vi "IOP Control.vi"() -> ()   [LabVIEW 2016]
uses:
  <vilib>/Platform/TimedLoop/XDataNode/timing_clust.ctl
  <vilib>/Platform/TimedLoop/XDataNode/nitl_modes.ctl
  <vilib>/Platform/TimedLoop/XDataNode/wakeup.ctl
  <vilib>/FPGAPlugInAG/PXI-7833R/niLvFpga_Open_PXI-7833R.vi
  <vilib>/Utility/error.llb/Error Cluster From Error Code.vi
  <vilib>/rvi/errors/niLvFpgaAdjustHostInterfaceError.vi
  <vilib>/Utility/file.llb/Write Delimited Spreadsheet (string).vi
  <vilib>/Utility/file.llb/Write Delimited Spreadsheet (DBL).vi
  Subsystems/Global Variables.vi
  <vilib>/FPGAPlugInAG/PXI-7833R/niLvFpga_Reset_PXI-7833R.vi
  <vilib>/FPGAPlugInAG/PXI-7833R/niLvFpga_Close_PXI-7833R.vi
  <vilib>/rvi/interface/nirviOpenFPGA/nirviOpenFPGA.xnode
  FPGA Bitfiles/PhantomControlPI_FPGATarget_QuadCtr2_E2412E44.lvbitx
  IRISS_FPGA_IO.vi
  <vilib>/rvi/interface/nirviReadWriteControl/nirviReadWriteControl.xnode
  <vilib>/platform/TimedLoop/XDataNode/XDataNode.xnode
  <vilib>/rvi/interface/nirviMethod/nirviMethod.xnode
  <vilib>/rvi/interface/nirviCloseFPGA/nirviCloseFPGA.xnode
  <vilib>/Platform/TimedLoop/XDataNode/XDNodeRunTimeDep.lvlib
  Library/KevinLibraryAll/labview2011/kevLib2011.lvlib
  NiFpgaLv.dll
panel:
  out "Pump Period":i32
  in  "Irr Cmd":sgl min=0 max=5 step=0.01 format="%#_4g"
  in  "Tab Control":T1(tab)
  in  "Pump PID Gains":cluster{"Kp":dbl, "Kd":dbl, "Ki":dbl, "Ts":dbl}={"Kp"=0.05, "Kd"=0.01, "Ki"=0.08, "Ts"=0.01}
  in  "Pump Ctrl":bool
  in  "IV Pole PID":cluster{"Kp":dbl, "Kd":dbl, "Ki":dbl, "Ts":dbl}={"Kp"=0.04, "Kd"=0.0, "Ki"=0.03, "Ts"=0.01}
  in  "IV Ctrl":bool
  in  "Pump PD":cluster{"Kp":dbl, "Kd":dbl, "Ki":dbl, "Ts":dbl}={"Kp"=0.001, "Kd"=0.0, "Ki"=0.001, "Ts"=0.01}
  in  "IV Pole PI":cluster{"Kp":dbl, "Kd":dbl, "Ki":dbl, "Ts":dbl}={"Kp"=0.04, "Kd"=0.0, "Ki"=0.03, "Ts"=0.01}
  in  "Dual Stage Ctrl":bool
  in  "Gen Filter":bool
  in  "Cutoff Freq":dbl=5.0 format="%#_13g"
  out "num_LP":dbl[](array[numeric])
  out "num_HP":dbl[](array[numeric])
  in  "Vac PID Gains":cluster{"Kp":dbl, "Kd":dbl, "Ki":dbl, "Ts":dbl}={"Kp"=5.0, "Kd"=0.0, "Ki"=5.0, "Ts"=0.01}
  in  "PID ON/OFF":bool
  in  "OCT Ctrl":bool
  in  "OCT Ctrl PI":cluster{"Kp":dbl, "Kd":dbl, "Ki":dbl, "Ts":dbl}={"Kp"=1.0, "Kd"=0.0, "Ki"=1.0, "Ts"=0.01}
  in  "Irr ON/OFF":bool
  out "Pressure Reading":dbl[](array[numeric]) caption="IOP Output [mmHg]"
  in  "Vacuum Step":bool
  in  "Increase":bool
  in  "Vac Step Size":sgl=50.0 min=0 max=100 step=1 format="%#_13g"
  in  "Wait Time [ms]":i32=200
  in  "Max Limit [mmHg]":dbl=600.0
  in  "Target IOP":sgl=20.0 min=0 max=100 step=1 format="%#_13g"
  out "Vac Input":sgl
  in  "Pump Max":dbl=5.0
  in  "Height":i32
  in  "IV Pole Max":dbl=95.0
  in  "Vac Cmd":sgl min=0 max=100 step=1 format="%#_13g"
  out "Vac Cmd Indicator":dbl
  out "Error(s) Out on Program End":errorcluster
  out "Elaspsed Time":dbl
  in  "File Path":path=path "C:/IOPData1.txt"
  in  "Take Data":bool
  out "File Exists":bool
  in  "Seconds of Data":dbl=30.0
  in  "Prog Stop":bool
  out "I/A and IOP Pressure":T2(graph)
  out "Vac Cmd Chart":sgl(graph)
  # "Irrigation"
  # "Vacuum"
  # "Ant. Chamber"
  # "Vitreous"
  # "Data Saving"
  # "Feedback Control"
  # "1. PID memory release or ramp out\n2. control action direction"
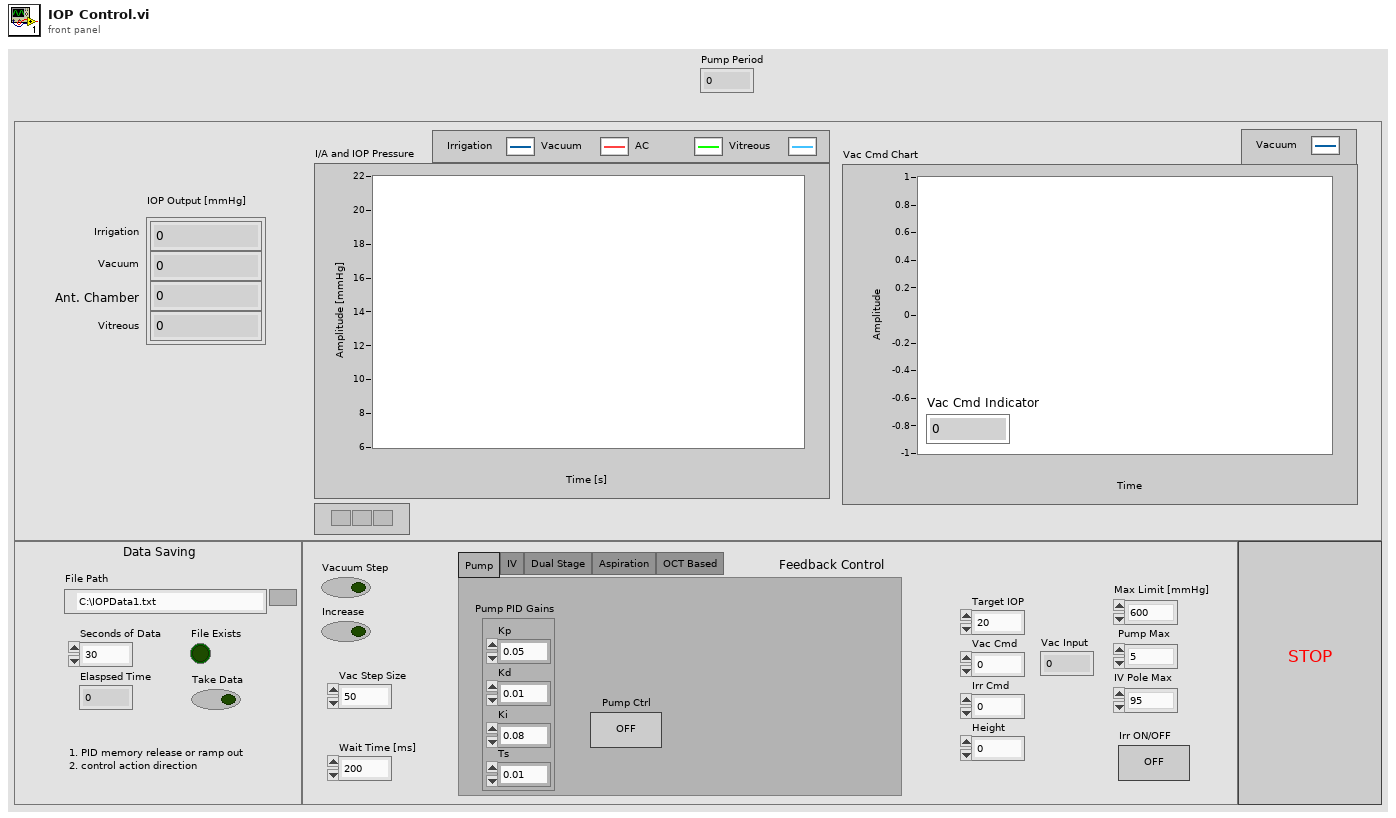
[diagram p1: front panel]
types:
  T1 = enum32{"Pump", "IV", "Dual Stage", "Aspiration", "OCT Based"}
  T2 = cluster{"[0]":dbl, "[1]":dbl, "[2]":dbl, "[3]":dbl, "[4]":dbl, "[5]":dbl, "[6]":dbl, "[7]":dbl, "[8]":dbl}
  T3 = typedef "XDNodeRunTimeDep.lvlib/timing_clust.ctl" = cluster{"Expected End [f-1]":u64, "Actual End [f-1]":u64, "Finished Late? [f-1]":bool, "Expected End [i-1]":u64, "Actual End [i-1]":u64, "Finished Late? [i-1]":bool, "Expected Start [i]":u64, "Actual Start [i]":u64, "Expected Start [f]":u64, "Actual Start [f]":u64, "Source Name":string, "Structure Name":string, "Period":i64, "Deadline":i64, "Offset":i64, "Start":i64, "Priority":i32, "Timeout":i32, "Mode":T4, "Wakeup Reason":T5, "Error":errorcluster, "Source Type":string, "Secondary Source Type":string, "Global End Time":u64, "Global Start Time":u64, "Frame Duration":u64, "Iteration Duration":u64, "Assigned CPU":i32, "I/O Scan Engine Mode":u32}
  T4 = typedef "XDNodeRunTimeDep.lvlib/nitl_modes.ctl" = enum32{"No Change", "Process missed periods, maintain original phase", "Discard missed periods, maintain original phase", "Process missed periods, ignore original phase", "Discard missed periods, ignore original phase"}
  T5 = typedef "XDNodeRunTimeDep.lvlib/wakeup.ctl" = enum32{"Normal", "Aborted", "Asynchronous wakeup", "Timing source error", "Timed loop error", "Timeout"}
  T6 = cluster{"Pressure Reading[0]":dbl, "Pressure Reading[1]":dbl, "Pressure Reading[2]":dbl, "Pressure Reading[3]":dbl, "Pressure Reading[4]":dbl, "Pressure Reading[5]":dbl, "Pressure Reading[6]":dbl, "Pressure Reading[7]":dbl, "Pressure Reading[8]":dbl}
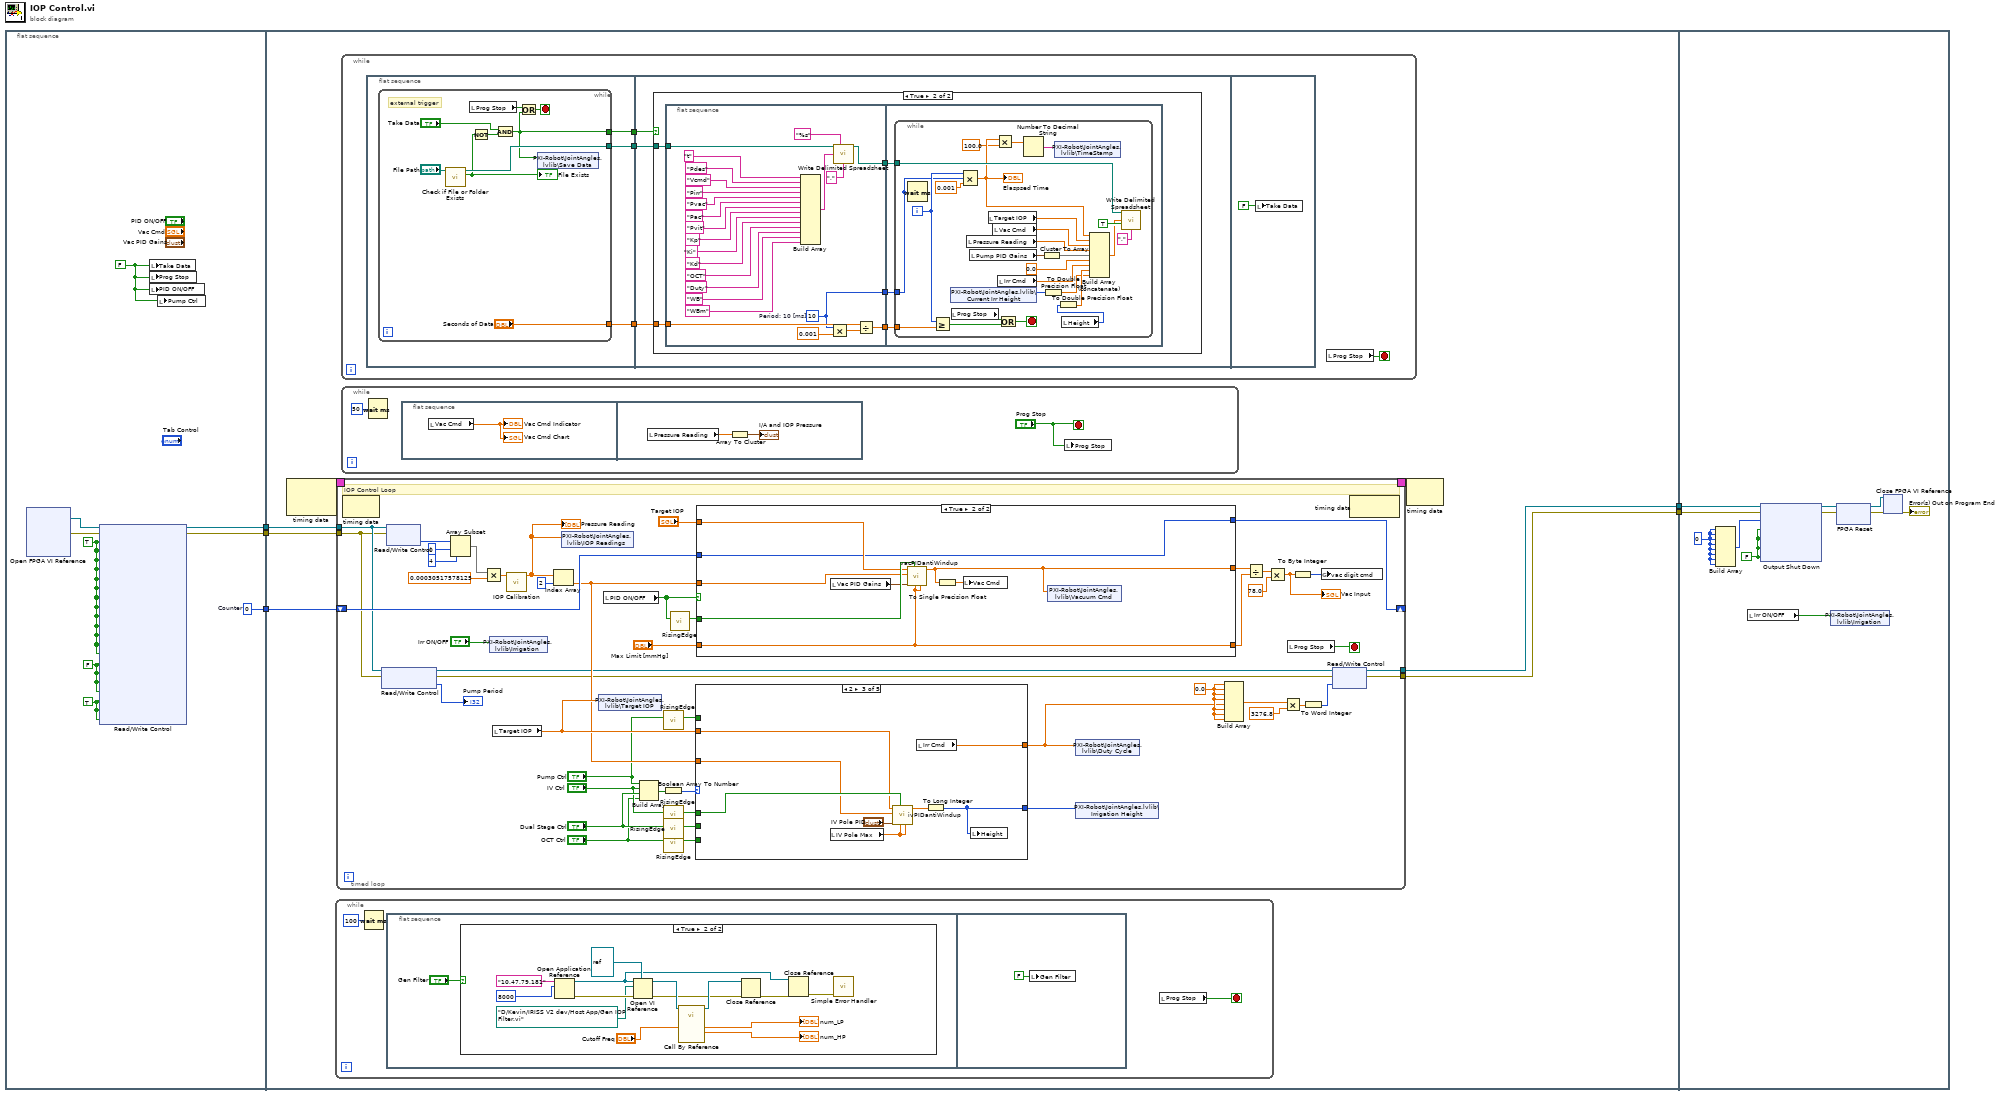
[diagram p0: block diagram]
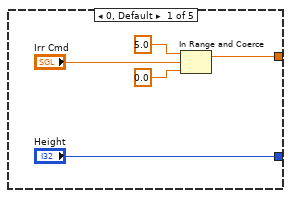
[diagram p3: hidden frame]
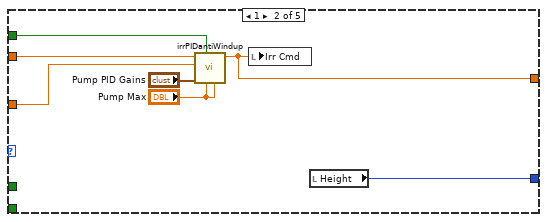
[diagram p4: hidden frame]
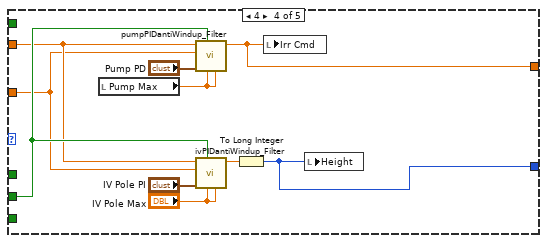
[diagram p5: hidden frame]
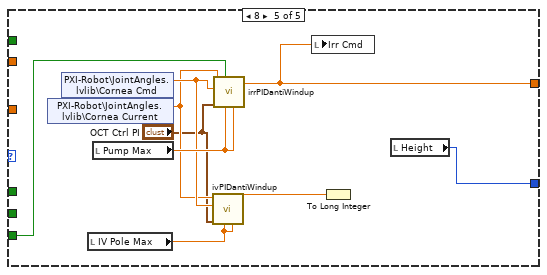
[diagram p6: hidden frame]
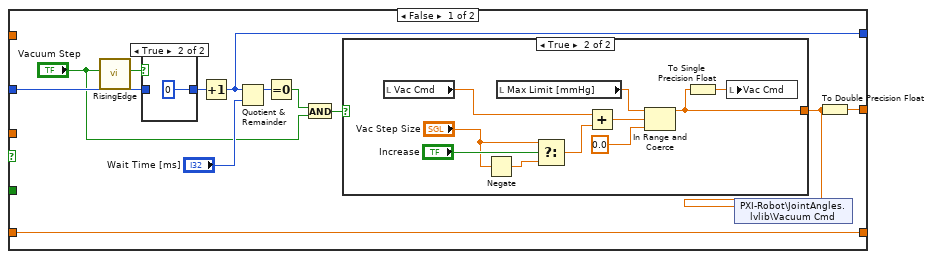
[diagram p7: hidden frame]
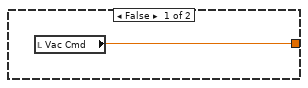
[diagram p9: hidden frame]
diagram:
  n1 = flat-sequence {
    tunnel: [w9] -> w5
    tunnel: [w8] -> w4
    tunnel: [w7] -> w3
    tunnel: w5 -> [w19]
    tunnel: w4 -> [w18]
    tunnel: w3 -> [w17]
    tunnel: [w16] -> w2
    tunnel: [w15] -> w1
    tunnel: w2 -> [w249]
    tunnel: w1 -> [w248]
    frame #0 {
      w7 = 0  # Counter
      w13 = TRUE ("Conn0/DIO12 Button 1")
      w12 = FALSE ("Reset")
      w14 = TRUE ("Reset")
      w6 = FALSE ("stop")
      n2 = xnode "Open FPGA VI Reference"() -> ("FPGA VI Reference Out"=w11:refnum<k20>, "error out"=w10:errorcluster)  [unwired: 2 in]
      n3 = xnode "Read/Write Control"("FPGA VI Reference In"=w11, "error in"=w10, "Reset 1"=w14, "Reset 3"=w14, "Reset 9"=w14, "Reset 10"=w14, "Reset 11"=w14, "Reset 12"=w14, "Reset 13"=w14, "Reset 14"=w14, "Reset 15"=w14, "Reset 16"=w14, "Reset 17"=w14, "Reset C1-1"=w14, "Reset C1-4"=w14, "INHB X"=w12, "INHB Y"=w12, "INHB Z"=w12, "INHB OCT Mot"=w12, "Conn0/DIO12 Button 1"=w13, "Conn0/DIO13 Button 2"=w13, "Conn0/DIO15 Button 4"=w13) -> ("FPGA VI Reference Out"=w9:refnum<k20>, "error out"=w8:errorcluster)
      n4 = local write "Take Data"(w6) -> ()
      n5 = local write "Prog Stop"(w6) -> ()
      n6 = local write "PID ON/OFF"(w6) -> ()
      n7 = local write "Pump Ctrl"(w6) -> ()
    }
    frame #1 {
      n8 = node-c288 ("Input Node")() -> (w21:T3)  [unwired: 2 in]
      n9 = while {
        stop <- w22 stop-if-true
        n10 = Wait (ms)(milliseconds to wait=u32 100) -> ()  [unwired: 1 out]
        n11 = flat-sequence {
          frame #0 {
            n12 = case shown="True" "Gen Filter" {
              frame False {
              }
              frame True {
                n13 = Open Application Reference(10:u16 8000 ("port number or service name (3363)"), 11:"10.47.79.181" ("machine name (\"\":  open local reference)")) -> (0:w33:errorcluster, 3:w35:refnum<vi>)  [unwired: 2 in]
                n14 = Open VI Reference(type specifier VI Refnum (for type only)=refnum<vi> refnum, application reference (local)=w35, vi path=path "D:/Kevin/IRISS V2 dev/Host App/Gen IOP Filter.vi", error in (no error)=w33) -> (vi reference=w30:refnum<vi>, error out=w28:errorcluster)  [unwired: 2 in]
                n15 = call-by-ref "?"(reference=w30, "Cutoff Freq"="Cutoff Freq") -> (reference out=w29:refnum<vi>, "num_HP"=→"num_HP":dbl[], "num_LP"=→"num_LP":dbl[])  [unwired: 10 in, 1 out]
                n16 = Close Reference(reference=w29, error in (no error)=w28) -> (error out=w34:errorcluster)
                n17 = Close Reference(reference=w35, error in (no error)=w34) -> (error out=w32:errorcluster)
                n18 = call <vilib>:"Simple Error Handler.vi"("error in (no error)"=w32) -> ()  [unwired: 4 in, 5 out]
              }
            }
          }
          frame #1 {
            n19 = local write "Gen Filter"(FALSE ("Gen Filter")) -> ()
          }
        }
        n20 = local read "Prog Stop"() -> (w22:bool)
      }
      n21 = timed-loop {
        timing: w21 -> [_]
        timing-out: [_] -> w20
        tunnel: w19 -> [w44]
        tunnel: w18 -> [w42]
        shift-right: [w68] -> _
        shift-left: w17 -> [w69]
        tunnel: [w67] -> w16
        tunnel: [w66] -> w15
        stop <- w79 stop-if-true
        w46 = 0.0 ("lower limit")
        # "IOP Control Loop"
        n22 = node-c288() -> ()  [unwired: 1 in, 1 out]
        n23 = xnode "Read/Write Control"("FPGA VI Reference In"=w44, "error in"=w42) -> ("FPGA VI Reference Out"=w43:refnum<k20>, "error out"=w41:errorcluster, "Pump Period"=→"Pump Period":i32)
        n24 = xnode "Read/Write Control"("FPGA VI Reference In"=w44, "error in"=w42) -> ("AI"=w82:i16[])  [unwired: 2 out]
        n25 = Array Subset(array=w82, index=0, length=4) -> (w87:i16[])
        n26 = Multiply(x=w87, y=0.00030517578125) -> (x*y=w72:dbl[])
        n27 = shared-variable "PXI-Robot\\JointAngles.lvlib\\Irrigation"("Irr ON/OFF") -> ()  [unwired: 1 in, 1 out]
        n28 = local read "Target IOP"() -> (w63:sgl)
        n29 = call "IOP Calibration.vi"("IOP Input [V]"=w72) -> ("IOP Output [mmHg]"=w64:dbl[])  [unwired: 10 in]
        "Pressure Reading" <- w64
        n30 = Index Array(array=w64, index=2) -> (element=w62:dbl)
        n31 = shared-variable "PXI-Robot\\JointAngles.lvlib\\IOP Readings"(w64) -> ()  [unwired: 1 in, 1 out]
        n32 = shared-variable "PXI-Robot\\JointAngles.lvlib\\Target IOP"(w63) -> ()  [unwired: 1 in, 1 out]
        n33 = local read "PID ON/OFF"() -> (w80:bool)
        n34 = Build Array("Pump Ctrl", "IV Ctrl", "Dual Stage Ctrl", "OCT Ctrl") -> (w59:bool[])
        n35 = call "RisingEdge.vi"("Signal In"="Pump Ctrl") -> ("Rising Edge"=w61:bool)  [unwired: 10 in]
        n36 = Boolean Array To Number(Boolean array=w59) -> (number=w60:u32)
        n37 = call "RisingEdge.vi"("Signal In"="IV Ctrl") -> ("Rising Edge"=w53:bool)  [unwired: 10 in]
        n38 = call "RisingEdge.vi"("Signal In"="Dual Stage Ctrl") -> ("Rising Edge"=w57:bool)  [unwired: 10 in]
        n39 = call "RisingEdge.vi"("Signal In"="OCT Ctrl") -> ("Rising Edge"=w51:bool)  [unwired: 10 in]
        n40 = call "RisingEdge.vi"("Signal In"=w80) -> ("Rising Edge"=w81:bool)  [unwired: 10 in]
        n41 = case shown="2" w60 {
          tunnel: w63 -> [_ w97 w106 w113 _]
          tunnel: w62 -> [_ w96 w105 w112 _]
          tunnel: w61 -> [_ w95 _ _ _]
          tunnel: [w88 w93 w100 w108 w118] -> w45
          tunnel: ["Height" w94 w101 w117 w119] -> w56
          tunnel: w57 -> [_ _ _ w114 _]
          tunnel: w53 -> [_ _ w107 _ _]
          tunnel: w51 -> [_ _ _ _ w125]
          frame 0, Default {
            n42 = In Range and Coerce(upper limit=5.0, x="Irr Cmd", lower limit=0.0) -> (coerced(x)=w88:dbl)  [unwired: 1 out]
          }
          frame 1 {
            n43 = call "irrPIDantiWindup.vi"("Saturation U"="Pump Max", "Saturation M"="Pump Max", "Reset"=w95, "PID Gains"="Pump PID Gains", "Feedback"=w96, "Reference"=w97) -> ("Control"=w93:dbl)  [unwired: 5 in]
            n44 = local write "Irr Cmd"(w93) -> ()
            n45 = local read "Height"() -> (w94:i32)
          }
          frame 2 {
            n46 = local read "IV Pole Max"() -> (w103:dbl)
            n47 = call "ivPIDantiWindup.vi"("Saturation U"=w103, "Saturation M"=w103, "Reset"=w107, "PID Gains"="IV Pole PID", "Feedback"=w105, "Reference"=w106) -> ("Control"=w102:dbl)  [unwired: 5 in]
            n48 = local read "Irr Cmd"() -> (w100:sgl)
            n49 = To Long Integer(number=w102) -> (32bit integer=w101:i32)
            n50 = local write "Height"(w101) -> ()
          }
          frame 4 {
            n51 = local read "Pump Max"() -> (w110:dbl)
            n52 = call "pumpPIDantiWindup_Filter.vi"("Saturation U"=w110, "Saturation M"=w110, "Reset"=w114, "PID Gains"="Pump PD", "Feedback"=w112, "Reference"=w113) -> ("Control"=w108:dbl)  [unwired: 5 in]
            n53 = call "ivPIDantiWindup_Filter.vi"("Saturation U"="IV Pole Max", "Saturation M"="IV Pole Max", "Reset"=w114, "PID Gains"="IV Pole PI", "Feedback"=w112, "Reference"=w113) -> ("Control"=w116:dbl)  [unwired: 5 in]
            n54 = To Long Integer(number=w116) -> (32bit integer=w117:i32)
            n55 = local write "Irr Cmd"(w108) -> ()
            n56 = local write "Height"(w117) -> ()
          }
          frame 8 {
            n57 = shared-variable "PXI-Robot\\JointAngles.lvlib\\Cornea Current"() -> (w123:dbl)  [unwired: 1 in, 1 out]
            n58 = shared-variable "PXI-Robot\\JointAngles.lvlib\\Cornea Cmd"() -> (w124:dbl)  [unwired: 1 in, 1 out]
            n59 = local read "IV Pole Max"() -> (w121:dbl)
            n60 = local read "Pump Max"() -> (w126:dbl)
            n61 = call "ivPIDantiWindup.vi"("Saturation U"=w121, "Saturation M"=w121, "PID Gains"="OCT Ctrl PI", "Feedback"=w124, "Reference"=w123) -> ("Control"=w120:dbl)  [unwired: 6 in]
            n62 = call "irrPIDantiWindup.vi"("Saturation U"=w126, "Saturation M"=w126, "Reset"=w125, "PID Gains"="OCT Ctrl PI", "Feedback"=w124, "Reference"=w123) -> ("Control"=w118:dbl)  [unwired: 5 in]
            n63 = local write "Irr Cmd"(w118) -> ()
            n64 = To Long Integer(number=w120) -> ()  [unwired: 1 out]
            n65 = local read "Height"() -> (w119:i32)
          }
        }
        n66 = case shown="True" w80 {
          tunnel: w62 -> [_ w156]
          tunnel: "Target IOP" -> [_ w157]
          tunnel: [w138 w152] -> w78
          tunnel: "Max Limit [mmHg]" -> [w137 w159]
          tunnel: [w137 w159] -> w70
          tunnel: w81 -> [_ w158]
          tunnel: w69 -> [w131 w153]
          tunnel: [w128 w153] -> w68
          frame False {
            n67 = call "RisingEdge.vi"("Signal In"="Vacuum Step") -> ("Rising Edge"=w132:bool)  [unwired: 10 in]
            n68 = case shown="True" w132 {
              tunnel: [w139 0] -> w135
              tunnel: w131 -> [w139 _]
              frame False {
              }
              frame True {
              }
            }
            n69 = Increment(x=w135) -> (x+1=w128:i32)
            n70 = Quotient & Remainder(x=w128, y="Wait Time [ms]") -> (x-y*floor(x/y)=w134:i32)  [unwired: 1 out]
            n71 = Equal To 0?(x=w134) -> (x = 0?=w136:bool)
            n72 = And(x=w136, y="Vacuum Step") -> (x .and. y?=w130:bool)
            n73 = case shown="True" w130 {
              tunnel: [w141 w151] -> w127
              frame False {
                n74 = local read "Vac Cmd"() -> (w141:sgl)
              }
              frame True {
                n75 = local read "Vac Cmd"() -> (w145:sgl)
                n76 = Negate(x="Vac Step Size") -> (-x=w143:sgl)
                n77 = local read "Max Limit [mmHg]"() -> (w148:dbl)
                n78 = Select(t="Vac Step Size", s="Increase", f=w143) -> (s? t:f=w146:sgl)
                n79 = Add(x=w145, y=w146) -> (x+y=w150:sgl)
                n80 = In Range and Coerce(upper limit=w148, x=w150, lower limit=0.0 ("y")) -> (coerced(x)=w151:dbl)  [unwired: 1 out]
                n81 = To Single Precision Float(number=w151) -> (single precision float=w142:sgl)
                n82 = local write "Vac Cmd"(w142) -> ()
              }
            }
            n83 = shared-variable "PXI-Robot\\JointAngles.lvlib\\Vacuum Cmd"(w127) -> ()  [unwired: 1 in, 1 out]
            n84 = To Double Precision Float(number=w127) -> (double precision float=w138:dbl)
          }
          frame True {
            n85 = local read "Vac PID Gains"() -> (w155:cluster{"Kp":dbl, "Kd":dbl, "Ki":dbl, "Ts":dbl})
            n86 = call "vacPIDantiWindup.vi"("Saturation U"=w159, "Saturation M"=w159, "Reset"=w158, "PID Gains"=w155, "Feedback"=w156, "Reference"=w157) -> ("Control"=w152:dbl)  [unwired: 5 in]
            n87 = To Single Precision Float(number=w152) -> (single precision float=w154:sgl)
            n88 = local write "Vac Cmd"(w154) -> ()
            n89 = shared-variable "PXI-Robot\\JointAngles.lvlib\\Vacuum Cmd"(w152) -> ()  [unwired: 1 in, 1 out]
          }
        }
        n90 = shared-variable "PXI-Robot\\JointAngles.lvlib\\Duty Cycle"(w45) -> ()  [unwired: 1 in, 1 out]
        n91 = shared-variable "PXI-Robot\\JointAngles.lvlib\\Irrigation Height"(w56) -> ()  [unwired: 1 in, 1 out]
        n92 = Build Array(w46, w46, w46, w46, w45, w46, w46, w46) -> (w47:dbl[])
        n93 = Divide(x=w78, y=w70) -> (x/y=w77:dbl)
        n94 = Multiply(x=w77, y=78.0) -> (x*y=w71:dbl)
        "Vac Input" <- w71
        n95 = Multiply(x=w47, y=3276.8) -> (x*y=w49:dbl[])
        n96 = local read "Prog Stop"() -> (w79:bool)
        n97 = To Byte Integer(number=w71) -> (8bit integer=w75:i8)
        n98 = To Word Integer(number=w49) -> (16bit integer=w48:i16[])
        n99 = global write "Global Variables.vi" "vac digit cmd"(w75) -> ()
        n100 = xnode "Read/Write Control"("FPGA VI Reference In"=w43, "error in"=w41, "AO"=w48) -> ("FPGA VI Reference Out"=w67:refnum<k20>, "error out"=w66:errorcluster)
        n101 = node-c288() -> ()  [unwired: 1 in, 1 out]
      }
      n102 = while {
        stop <- w169 stop-if-true
        n103 = flat-sequence {
          tunnel: [w173] -> w172
          tunnel: [w175] -> w171
          tunnel: [w174] -> w170
          tunnel: w172 -> [w187]
          tunnel: w171 -> [w186]
          tunnel: w170 -> [w185]
          frame #0 {
            n104 = while {
              tunnel: [w180] -> w175
              tunnel: ["Seconds of Data"] -> w174
              tunnel: [w176] -> w173
              stop <- w184 stop-if-true
              # "external trigger"
              n105 = call <vilib>:"Check if File or Folder Exists.vi"("path"="File Path") -> ("file or folder exists?"=w179:bool, "dup path"=w180:path)  [unwired: 8 in, 1 out]
              "File Exists" <- w179
              n106 = local read "Prog Stop"() -> (w182:bool)
              n107 = Not(x=w179) -> (.not. x?=w178:bool)
              n108 = And(x="Take Data", y=w178) -> (x .and. y?=w176:bool)
              n109 = Or(x=w182, y=w176) -> (x .or. y?=w184:bool)
              n110 = shared-variable "PXI-Robot\\JointAngles.lvlib\\Save Data"(w176) -> ()  [unwired: 1 in, 1 out]
            }
          }
          frame #1 {
            n111 = case shown="True" w187 {
              tunnel: w186 -> [_ w192]
              tunnel: w185 -> [_ w190]
              frame False {
              }
              frame True {
                n112 = flat-sequence {
                  tunnel: w192 -> [w206]
                  tunnel: [w204] -> w191
                  tunnel: w190 -> [w214]
                  tunnel: [w212] -> w189
                  tunnel: [w201] -> w188
                  tunnel: w191 -> [w219]
                  tunnel: w189 -> [w218]
                  tunnel: w188 -> [w217]
                  frame #0 {
                    w201 = 10  # Period: 10 [ms]
                    n113 = Build Array("t" ("delimiter (\\t)"), "Pdes" ("delimiter (\\t)"), "Vcmd" ("delimiter (\\t)"), "Pirr" ("delimiter (\\t)"), "Pvac" ("delimiter (\\t)"), "Pac" ("delimiter (\\t)"), "Pvit" ("delimiter (\\t)"), "Kp" ("delimiter (\\t)"), "Ki" ("delimiter (\\t)"), "Kd" ("delimiter (\\t)"), "OCT" ("delimiter (\\t)"), "Duty" ("delimiter (\\t)"), "WB" ("delimiter (\\t)"), "WBm" ("delimiter (\\t)")) -> (w203:string[])
                    n114 = Multiply(x=w201, y=0.001) -> (x*y=w213:dbl)
                    n115 = call-poly <vilib>:"Write Delimited Spreadsheet.vi"("file path (dialog if empty)"=w206, "format (%s)"="%s", "1D data"=w203, "delimiter (\\t)"="," ("delimiter (\\t)")) -> ("new file path (Not A Path if cancelled)"=w204:path)  [unwired: 10 in, 1 out]
                    n116 = Divide(x=w214, y=w213) -> (x/y=w212:dbl)
                  }
                  frame #1 {
                    n117 = while {
                      tunnel: w219 -> [w239]
                      tunnel: w218 -> [w241]
                      tunnel: w217 -> [w232]
                      i -> [w242]
                      stop <- w244 stop-if-true
                      n118 = Wait (ms)(milliseconds to wait=w232) -> ()  [unwired: 1 out]
                      n119 = Greater Or Equal?(x=w242, y=w241) -> (x >= y?=w240:bool)
                      n120 = shared-variable "PXI-Robot\\JointAngles.lvlib\\Current Irr Height"() -> (w231:i32)  [unwired: 1 in, 1 out]
                      n121 = local read "Prog Stop"() -> (w245:bool)
                      n122 = Compound Arithmetic op=MULTIPLY(w242, w232, 0.001 ("y")) -> (w226:dbl)
                      "Elaspsed Time" <- w226
                      n123 = local read "Pressure Reading"() -> (w233:dbl[])
                      n124 = local read "Pump PID Gains"() -> (w221:cluster{"Kp":dbl, "Kd":dbl, "Ki":dbl, "Ts":dbl})
                      n125 = local read "Target IOP"() -> (w235:sgl)
                      n126 = local read "Vac Cmd"() -> (w234:sgl)
                      n127 = Multiply(x=w226, y=100.0) -> (x*y=w224:dbl)
                      n128 = local read "Irr Cmd"() -> (w222:sgl)
                      n129 = Or(x=w245, y=w240) -> (x .or. y?=w244:bool)
                      n130 = Number To Decimal String(number=w224) -> (decimal integer string=w223:string)  [unwired: 1 in]
                      n131 = Cluster To Array(cluster=w221) -> (array=w220:dbl[])
                      n132 = To Double Precision Float(number=w231) -> (double precision float=w227:dbl)
                      n133 = shared-variable "PXI-Robot\\JointAngles.lvlib\\TimeStamp"(w223) -> ()  [unwired: 1 in, 1 out]
                      n134 = local read "Height"() -> (w229:i32)
                      n135 = To Double Precision Float(number=w229) -> (double precision float=w228:dbl)
                      n136 = Build Array (concatenate)(w226, w235, w234, w233, w220, 0.0 ("y"), w222, w228, w227) -> (w237:dbl[])
                      n137 = call-poly <vilib>:"Write Delimited Spreadsheet.vi"("file path (dialog if empty)"=w239, "1D data"=w237, "append to file? (new file:F)"=TRUE, "delimiter (\\t)"="," ("delimiter (\\t)")) -> ()  [unwired: 10 in, 2 out]
                    }
                  }
                }
              }
            }
          }
          frame #2 {
            n138 = local write "Take Data"(FALSE) -> ()
          }
        }
        n139 = local read "Prog Stop"() -> (w169:bool)
      }
      n140 = while {
        stop <- "Prog Stop" stop-if-true
        n141 = Wait (ms)(milliseconds to wait=u32 50) -> ()  [unwired: 1 out]
        n142 = flat-sequence {
          frame #0 {
            n143 = local read "Vac Cmd"() -> (→"Vac Cmd Chart" →"Vac Cmd Indicator":sgl)
          }
          frame #1 {
            n144 = local read "Pressure Reading"() -> (w168:dbl[])
            n145 = Array To Cluster(array=w168) -> (cluster=→"I/A and IOP Pressure":T6)
          }
        }
        n146 = local write "Prog Stop"("Prog Stop") -> ()
      }
      n147 = node-c288(w20) -> ()  [unwired: 1 out]
    }
    frame #2 {
      w252 = FALSE
      w254 = i16 0 ("element")
      n148 = Build Array(w254, w254, w254, w254, w254, w254, w254, w254) -> (w253:i16[])
      n149 = local read "Irr ON/OFF"() -> (w247:bool)
      n150 = xnode "Output Shut Down"("FPGA VI Reference In"=w249, "error in"=w248, "AO"=w253, "INHB X"=w252, "INHB Y"=w252, "INHB Z"=w252, "INHB OCT Mot"=w252) -> ("FPGA VI Reference Out"=w251:refnum<k20>, "error out"=w250:errorcluster)
      n151 = shared-variable "PXI-Robot\\JointAngles.lvlib\\Irrigation"(w247) -> ()  [unwired: 1 in, 1 out]
      n152 = xnode "FPGA Reset"("FPGA VI Reference In"=w251, "error in"=w250) -> ("FPGA VI Reference Out"=w257:refnum<k20>, "error out"=w256:errorcluster)
      n153 = xnode "Close FPGA VI Reference"("FPGA VI Reference In"=w257, "error in"=w256) -> ("error out"=→"Error(s) Out on Program End":errorcluster)
    }
  }
